vi "niFPGA Friction_m.vi"   [LabVIEW 2017]
doc: "Implements a discontinuity at zero with linear behavior elsewhere. The data type you wire to <B>input</B> determines the <B>output</B> data type."
uses:
  <vilib>/rvi/Analysis/common/FxpNativeNode/niFpgaFxpNative.xnode
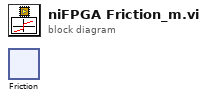
[diagram p0: block diagram]
diagram:
  n1 = xnode "Friction"() -> ()  [unwired: 3 in, 1 out]
